vi "XML - Update Mappings.vi"(6 "Channel Data in":T2 {"Dependent Node References" format="%.0x"}, 7 "Channel Path":string, 8 "error in (no error)":errorcluster, 9 "Channel Path Destinations":string[](array[string]), 10 "Channel Path Sources":string[](array[string]), 11 "Item Ref in":T1 format="%.0x") -> (0 "error out":errorcluster, 3 "Channel Data out":T2 {"Dependent Node References" format="%.0x"})   [LabVIEW 2019]
uses:
  <vilib>/NI VeriStand/Custom Device API/Custom Device Item Ref.ctl
  UDP-Custom-Device System Explorer.lvlib
  <vilib>/NI VeriStand/Custom Device API/Custom Device API.lvlib
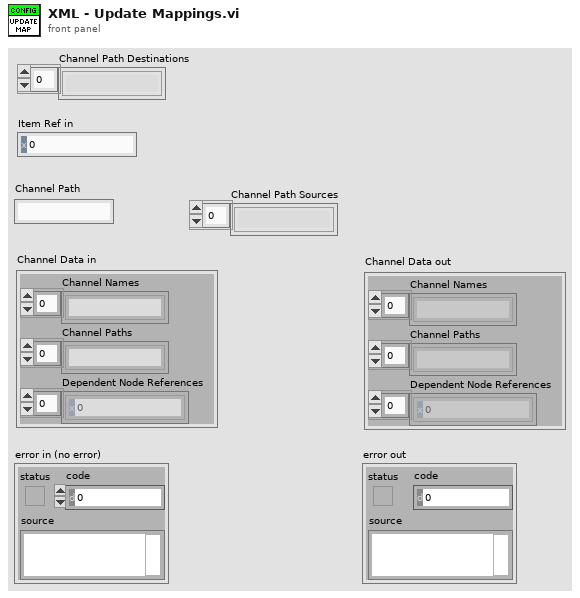
[diagram p1: front panel]
types:
  T1 = typedef "Custom Device API.lvlib/Custom Device Item Ref.ctl" = u64
  T2 = cluster{"Channel Names":string[], "Channel Paths":string[], "Dependent Node References":T1[]}
  T3 = typedef "Custom Device API.lvlib/Custom Device Item Info.ctl" = cluster{"Name":string, "Is Channel":bool, "GUID":string, "Is Waveform":bool}
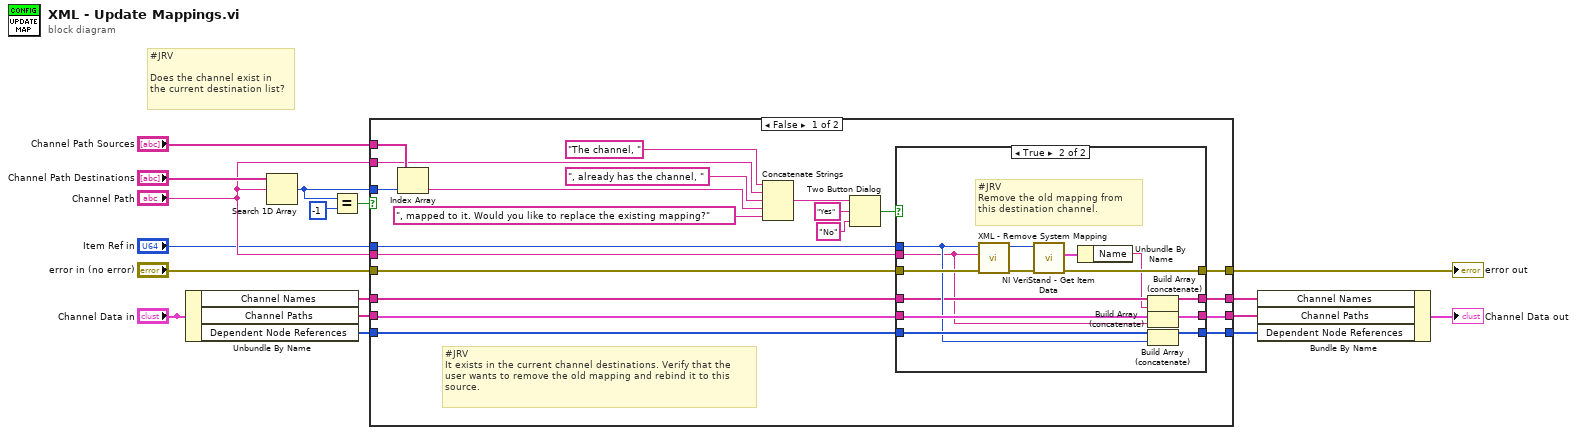
[diagram p0: block diagram]
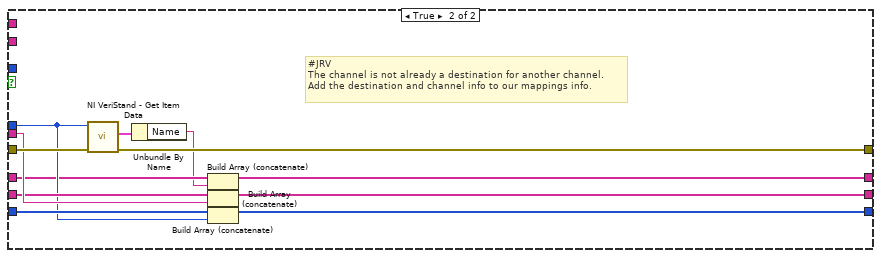
[diagram p3: hidden frame]
diagram:
  # "#JRV\n\nDoes the channel exist in\nthe current destination list?"
  n1 = Unbundle By Name("Channel Data in") -> ("Channel Names"=w12:string[], "Channel Paths"=w11:string[], "Dependent Node References"=w10:T1[])
  n2 = Search 1D Array(1D array="Channel Path Destinations", element="Channel Path") -> (index of element=w13:i32)  [unwired: 1 in]
  n3 = Equal?(x=w13, y=-1) -> (x = y?=w15:bool)
  n4 = case shown="False" w15 {
    tunnel: "Channel Path Sources" -> [w38 _]
    tunnel: w13 -> [w37 _]
    tunnel: "Channel Path" -> [w34 _]
    tunnel: w12 -> [w28 w59]
    tunnel: w11 -> [w26 w63]
    tunnel: w10 -> [w25 w62]
    tunnel: "Item Ref in" -> [w24 w61]
    tunnel: "Channel Path" -> [w23 w64]
    tunnel: "error in (no error)" -> [w22 w67]
    tunnel: [w21 w65] -> w9
    tunnel: [w20 w57] -> w8
    tunnel: [w19 w60] -> w7
    tunnel: [w18 w66] -> w5
    frame False {
      # "#JRV\nIt exists in the current channel destinations. Verify that the\nuser wants to remove the old mapping and rebind it to this\nsource."
      n5 = Index Array(array=w38, index=w37) -> (element=w33:string)
      n6 = Concatenate Strings("The channel, " ("Path"), w34, ", already has the channel, " ("Path"), w33, ", mapped to it. Would you like to replace the existing mapping?" ("Path")) -> (w31:string)
      n7 = Two Button Dialog(message=w31, 1:"No" ("F button name (\"Cancel\")"), 2:"Yes" ("T button name (\"OK\")")) -> (T button?=w27:bool)
      n8 = case shown="True" w27 {
        tunnel: w28 -> [w42 w48]
        tunnel: w26 -> [w41 w45]
        tunnel: w25 -> [w40 w51]
        tunnel: w24 -> [_ w50]
        tunnel: w23 -> [_ w44]
        tunnel: w22 -> [w39 w56]
        tunnel: [w42 w46] -> w21
        tunnel: [w41 w43] -> w20
        tunnel: [w40 w49] -> w19
        tunnel: [w39 w52] -> w18
        frame False {
          # "#JRV\nKeep the old binding."
        }
        frame True {
          # "#JRV\nRemove the old mapping from\nthis destination channel."
          n9 = call "XML - Remove System Mapping.vi"("error in (no error)"=w56, "Channel Path Destination"=w44, "Item Ref in"=w50) -> ("error out"=w55:errorcluster, "Item Ref out"=w54:T1)  [unwired: 7 in]
          n10 = call <vilib>:"NI VeriStand - Get Item Data.vi"("error in (no error)"=w55, "Item Ref in"=w54) -> ("error out"=w52:errorcluster, "Item Info"=w53:T3)  [unwired: 6 in, 2 out]
          n11 = Unbundle By Name(w53) -> ("Name"=w47:string)
          n12 = Build Array (concatenate)(w48, w47) -> (w46:string[])
          n13 = Build Array (concatenate)(w45, w44) -> (w43:string[])
          n14 = Build Array (concatenate)(w51, w50) -> (w49:T1[])
        }
      }
    }
    frame True {
      # "#JRV\nThe channel is not already a destination for another channel.\nAdd the destination and channel info to our mappings info."
      n15 = call <vilib>:"NI VeriStand - Get Item Data.vi"("error in (no error)"=w67, "Item Ref in"=w61) -> ("error out"=w66:errorcluster, "Item Info"=w68:T3)  [unwired: 6 in, 2 out]
      n16 = Unbundle By Name(w68) -> ("Name"=w58:string)
      n17 = Build Array (concatenate)(w59, w58) -> (w65:string[])
      n18 = Build Array (concatenate)(w63, w64) -> (w57:string[])
      n19 = Build Array (concatenate)(w62, w61) -> (w60:T1[])
    }
  }
  "error out" <- w5
  n20 = Bundle By Name(cluster="Channel Data in", "Channel Names"=w9, "Channel Paths"=w8, "Dependent Node References"=w7) -> (→"Channel Data out":T2)
